vi "Display_data.vi"() -> ()   [LabVIEW 2016]
uses:
  <vilib>/Utility/file.llb/Read Delimited Spreadsheet (DBL).vi
panel:
  in  "Ring":u16(ring) items=["Default", "Number Filter", "Average", "Integrate", "Derivate", "g"]
  in  "String":string
  out "Waveform Graph 2":dbl[](graph)
  out "Array":dbl[](array[numeric])
  in  "X vector":i32
  out "XY Graph":cluster{dbl[], "all rows":dbl[]}[](graph)
  in  "Inoput":dbl=15.0 format="%#_13g"
  in  "index (row) 3":i32
  in  "index (row) 2":i32
  in  "index (row)":i32
  out "all rows":dbl[][](array[numeric])
  out "Raw Data":dynamicdata(graph)
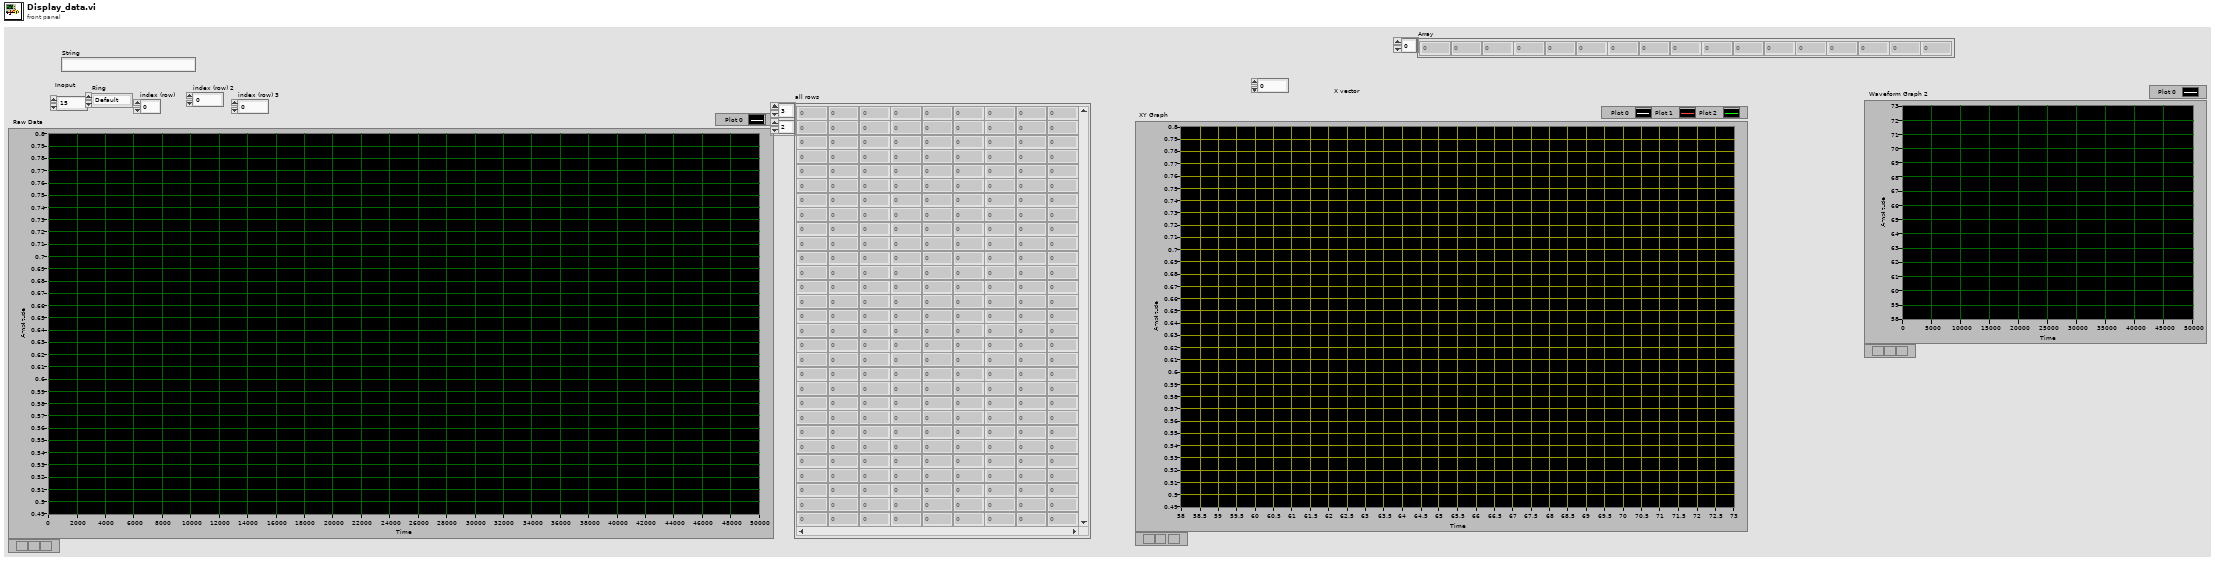
[diagram p1: front panel]
types:
  T1 = cluster{"Output Array":dbl[], "Output Array":dbl[]}
  T2 = cluster{"Output Array":dbl[], "Output Array":dbl[]}[]
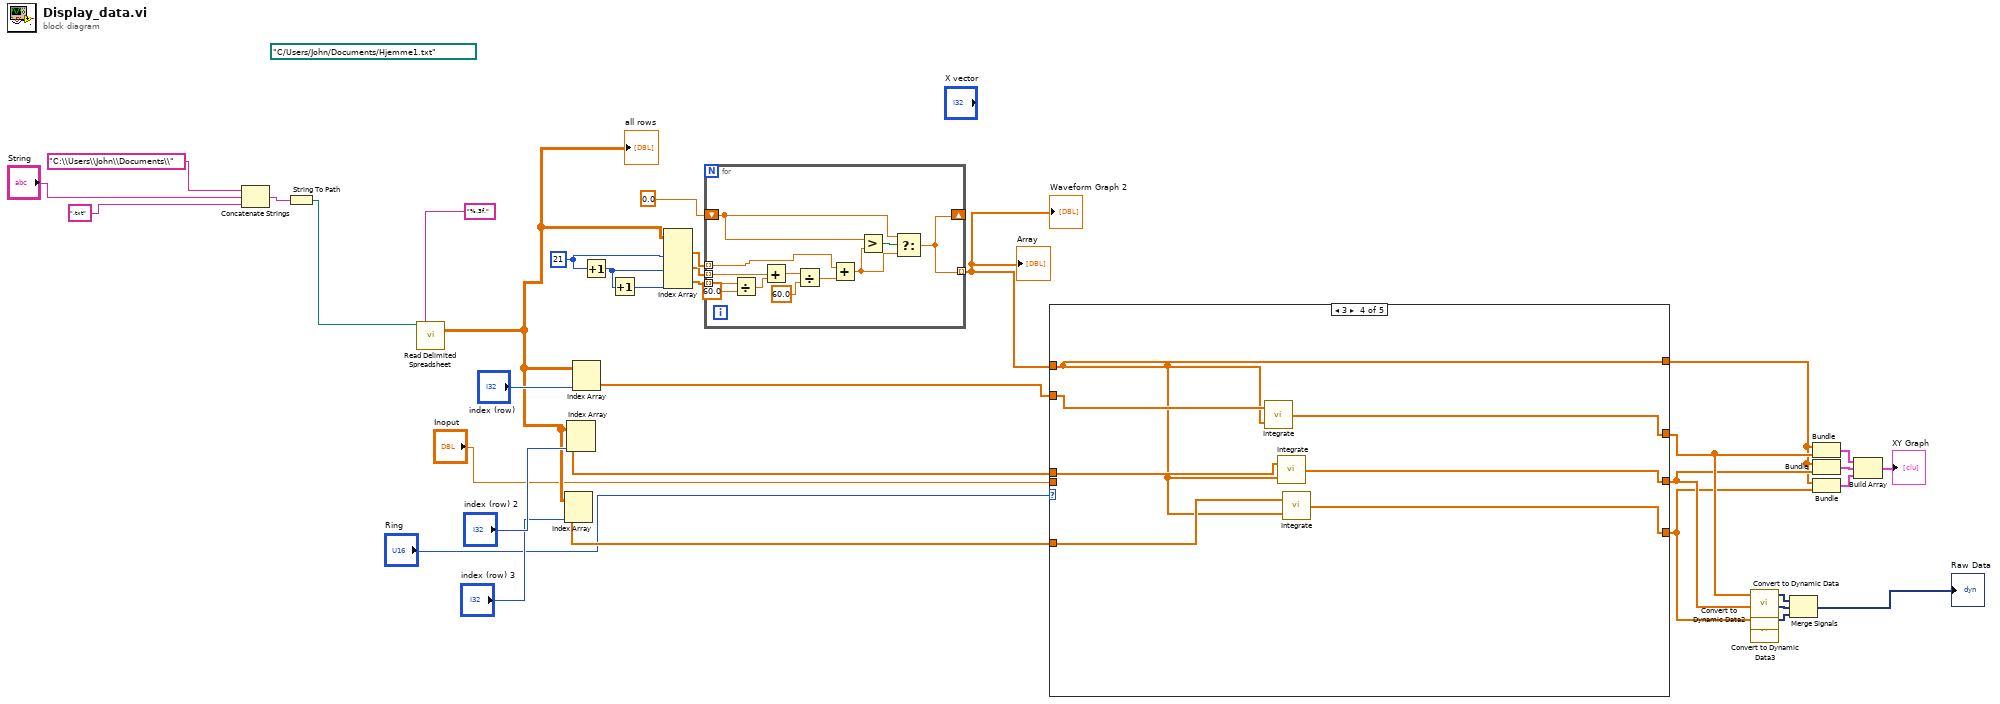
[diagram p0: block diagram]
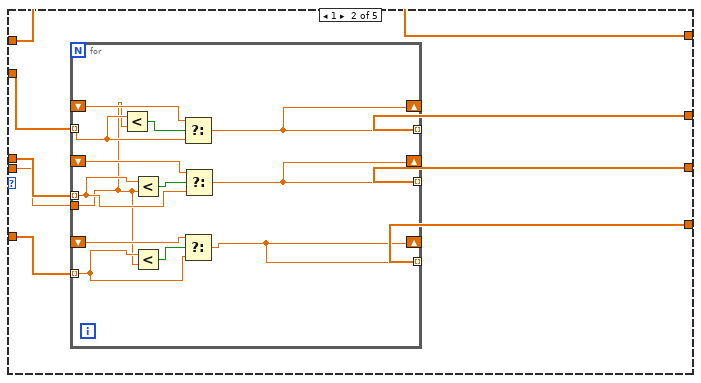
[diagram p3: hidden frame]
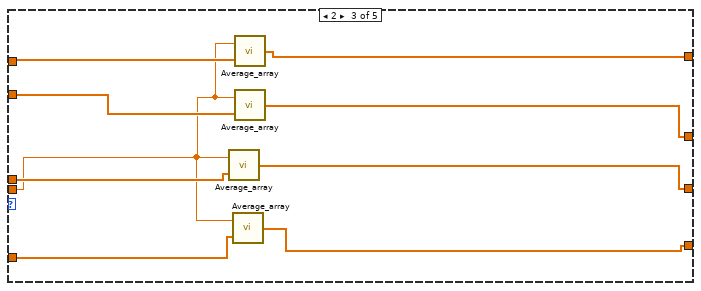
[diagram p4: hidden frame]
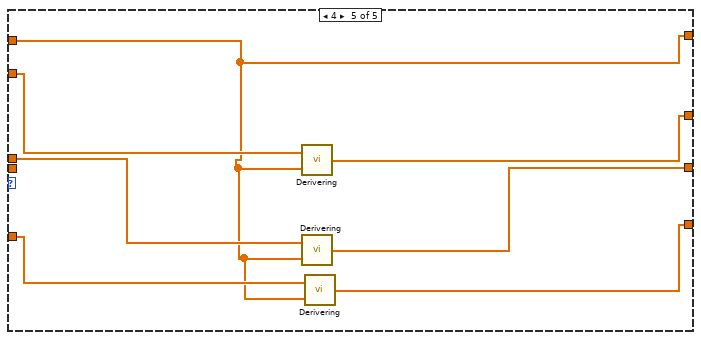
[diagram p5: hidden frame]
diagram:
  w23 = 21 ("index (col)")
  (unwired) path "C:/Users/John/Documents/Hjemme1.txt" ("file path (dialog if empty)")
  n1 = Concatenate Strings("C:\\Users\\John\\Documents\\", "String", ".txt") -> (w15:string)
  n2 = String To Path(string=w15) -> (path=w11:path)
  n3 = call-poly <vilib>:"Read Delimited Spreadsheet.vi"("file path (dialog if empty)"=w11, "format (%.3f)"="%.3f,") -> ("all rows"=w24:dbl[][])  [unwired: 8 in, 5 out]
  "all rows" <- w24
  n4 = Index Array(array=w24, index (col)="index (row) 3") -> (element=w25:dbl[])  [unwired: 1 in]
  n5 = Index Array(array=w24, index (col)="index (row) 2") -> (element=w26:dbl[])  [unwired: 1 in]
  n6 = Index Array(array=w24, index (col)="index (row)") -> (element=w27:dbl[])  [unwired: 1 in]
  n7 = Increment(x=w23) -> (x+1=w18:i32)
  n8 = Increment(x=w18) -> (x+1=w22:i32)
  n9 = Index Array(array=w24, index (col) #1=w23, index (col) #2=w18, index (col) #3=w22) -> (element #1=w21:dbl[], element #2=w20:dbl[], element #3=w19:dbl[])  [unwired: 3 in]
  n10 = for {
    tunnel: w21 -> [w39] mode=indexing
    tunnel: w20 -> [w41] mode=indexing
    tunnel: w19 -> [w40] mode=indexing
    tunnel: [w38] -> w2 mode=indexing
    shift-right: [w38] -> _
    shift-left: 0.0 -> [w37]
    n11 = Divide(x=w40, y=60.0) -> (x/y=w47:dbl)
    n12 = Add(x=w41, y=w47) -> (x+y=w42:dbl)
    n13 = Divide(x=w42, y=60.0) -> (x/y=w46:dbl)
    n14 = Add(x=w39, y=w46) -> (x+y=w36:dbl)
    n15 = Greater?(x=w37, y=w36) -> (0:w43:bool)
    n16 = Select(t=w37, s=w43, f=w36) -> (s? t:f=w38:dbl)
  }
  "Array" <- w2
  "Waveform Graph 2" <- w2
  n17 = case shown="3" "Ring" {
    tunnel: w27 -> [w51 w59 w79 w86 w95]
    tunnel: w26 -> [w50 w58 w80 w87 w94]
    tunnel: w25 -> [w49 w57 w81 w88 w93]
    tunnel: [w49 w56 w76 w83 w92] -> w9
    tunnel: [w50 w55 w77 w84 w91] -> w10
    tunnel: [w51 w54 w78 w85 w90] -> w17
    tunnel: "Inoput" -> [_ w53 w74 _ _]
    tunnel: w2 -> [w48 w52 w75 w82 w89]
    tunnel: [w48 w52 w73 w82 w89] -> w1
    frame 0, Default {
    }
    frame 1 {
      n18 = for {
        tunnel: w59 -> [w70] mode=indexing
        tunnel: w58 -> [w67] mode=indexing
        tunnel: w57 -> [w64] mode=indexing
        shift-right: [w61] -> _
        shift-left: _ -> [w62]
        shift-right: [w66] -> _
        shift-left: _ -> [w65]
        shift-right: [w72] -> _
        shift-left: _ -> [w71]
        tunnel: [w72] -> w54 mode=indexing
        tunnel: [w66] -> w55 mode=indexing
        tunnel: [w61] -> w56 mode=indexing
        tunnel: w53 -> [w60]
        n19 = Less?(x=w70, y=w60) -> (x < y?=w69:bool)
        n20 = Less?(x=w67, y=w60) -> (x < y?=w68:bool)
        n21 = Less?(x=w64, y=w60) -> (x < y?=w63:bool)
        n22 = Select(t=w71, s=w69, f=w70) -> (s? t:f=w72:dbl)
        n23 = Select(t=w62, s=w63, f=w64) -> (s? t:f=w61:dbl)
        n24 = Select(t=w65, s=w68, f=w67) -> (s? t:f=w66:dbl)
      }
    }
    frame 2 {
      n25 = call "Average_array.vi"("Input Array"=w80, "Average over.."=w74) -> ("Output Array"=w77:dbl[])
      n26 = call "Average_array.vi"("Input Array"=w81, "Average over.."=w74) -> ("Output Array"=w76:dbl[])
      n27 = call "Average_array.vi"("Input Array"=w75, "Average over.."=w74) -> ("Output Array"=w73:dbl[])
      n28 = call "Average_array.vi"("Input Array"=w79, "Average over.."=w74) -> ("Output Array"=w78:dbl[])
    }
    frame 3 {
      n29 = call "Integrate.vi"("Input Array Y"=w82, "Input Array X"=w86) -> ("Output Array"=w85:dbl[])
      n30 = call "Integrate.vi"("Input Array Y"=w82, "Input Array X"=w87) -> ("Output Array"=w84:dbl[])
      n31 = call "Integrate.vi"("Input Array Y"=w82, "Input Array X"=w88) -> ("Output Array"=w83:dbl[])
    }
    frame 4 {
      n32 = call "Derivering.vi"("Input Array Y"=w89, "Input Array X"=w95) -> ("Output Array"=w90:dbl[])
      n33 = call "Derivering.vi"("Input Array Y"=w89, "Input Array X"=w94) -> ("Output Array"=w91:dbl[])
      n34 = call "Derivering.vi"("Input Array Y"=w89, "Input Array X"=w93) -> ("Output Array"=w92:dbl[])
    }
  }
  n35 = call "Convert to Dynamic Data"("Array"=w17) -> ("Dynamic Data Type"=w31:dynamicdata)  [unwired: 3 in]
  n36 = call "Convert to Dynamic Data2"("Array"=w10) -> ("Dynamic Data Type"=w30:dynamicdata)  [unwired: 3 in]
  n37 = call "Convert to Dynamic Data3"("Array"=w9) -> ("Dynamic Data Type"=w29:dynamicdata)  [unwired: 3 in]
  n38 = Merge Signals(w31, w30, w29) -> (→"Raw Data":dynamicdata)
  n39 = Bundle("Output Array"=w1, "Output Array"=w17) -> (w8:T1)  [unwired: 1 in]
  n40 = Bundle("Output Array"=w1, "Output Array"=w10) -> (w7:T1)  [unwired: 1 in]
  n41 = Bundle("Output Array"=w1, "Output Array"=w9) -> (w6:T1)  [unwired: 1 in]
  n42 = Build Array(w8, w7, w6) -> (→"XY Graph":T2)
